vi "Set Attenuation.vi"(8 "error in (no error)":errorcluster, 10 "Attenuation":dbl, 11 "EXFO in":refnum<class "EXFO.lvclass">) -> (0 "error out":errorcluster, 3 "EXFO out":refnum<class "EXFO.lvclass">)   [LabVIEW 2018, in "EXFO.lvlib" / "EXFO.lvclass"]
doc: "This is a dynamically dispatched VI. The child method will use the appropriate protocols to set the attenuation level on the Variable Optical Attenuator. Additionally, the parent method records the set attenuation value.\n\nAuthor: Ron Dexter\nCompany: Luminar\nModified: 5/20/2018"
uses:
  EXFO.lvclass
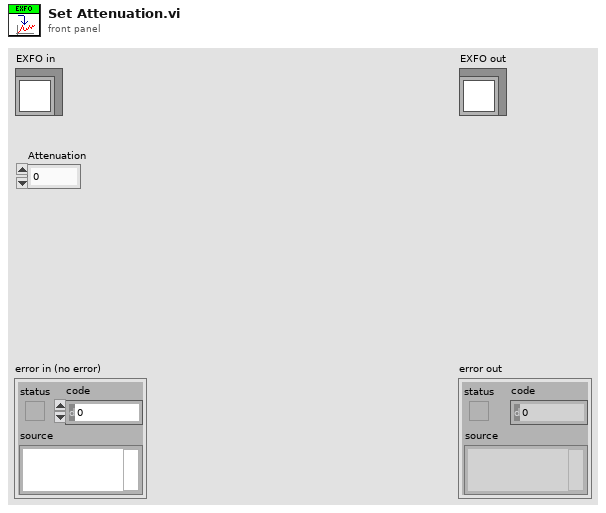
[diagram p1: front panel]
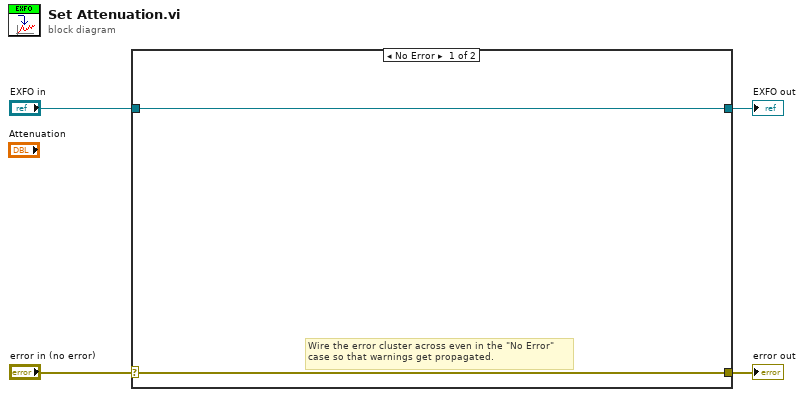
[diagram p0: block diagram]
diagram:
  n1 = case shown="No Error" "error in (no error)" {
    selector: "error in (no error)" -> [w6 w8]
    tunnel: [w6 w8] -> w3
    tunnel: [w5 w7] -> w1
    tunnel: "EXFO in" -> [w5 w7]
    frame No Error {
      # "Wire the error cluster across even in the \"No Error\"\ncase so that warnings get propagated."
    }
    frame Error {
    }
  }
  "error out" <- w3
  "EXFO out" <- w1
